vi "Dual_Joy_Combine.vi"(0 "Joy1":dbl, 1 "Joy2":dbl, 3 "Z":bool) -> (7 "Output":dbl)   [LabVIEW 2017]
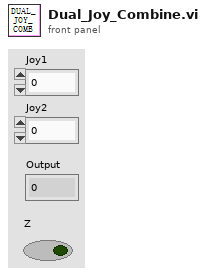
[diagram p1: front panel]
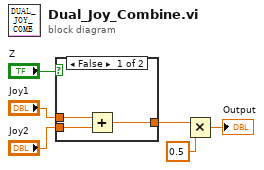
[diagram p0: block diagram]
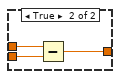
[diagram p2: hidden frame]
diagram:
  n1 = case shown="False" "Z" {
    tunnel: "Joy1" -> [w8 w12]
    tunnel: "Joy2" -> [w9 w11]
    tunnel: [w7 w10] -> w1
    frame False {
      n2 = Add(x=w8, y=w9) -> (x+y=w7:dbl)
    }
    frame True {
      n3 = Subtract(x=w12, y=w11) -> (x-y=w10:dbl)
    }
  }
  n4 = Multiply(x=w1, y=0.5) -> (x*y=→"Output":dbl)
